vi "AVL Auto Time v0.1.vi"(9 "Time of Exit in":timestamp, 10 "Non-Auto Time in":dbl, 11 "State":T1) -> (2 "Time of Exit":timestamp, 3 "Non-Auto Time":dbl)   [LabVIEW 2021]
doc: "v0.1:\n- Added a state to reload values"
uses:
  Controls/AVL Auto Time.ctl
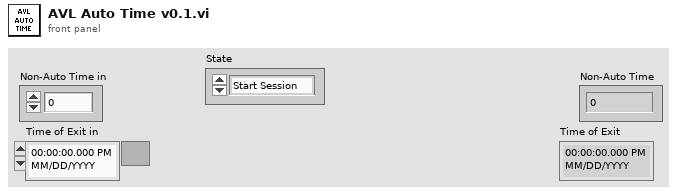
[diagram p1: front panel]
types:
  T1 = typedef "AVL Auto Time.ctl" = enum16{"Start Session", "Exited Auto", "Resumed Auto", "Read Time", "Reload Values"}
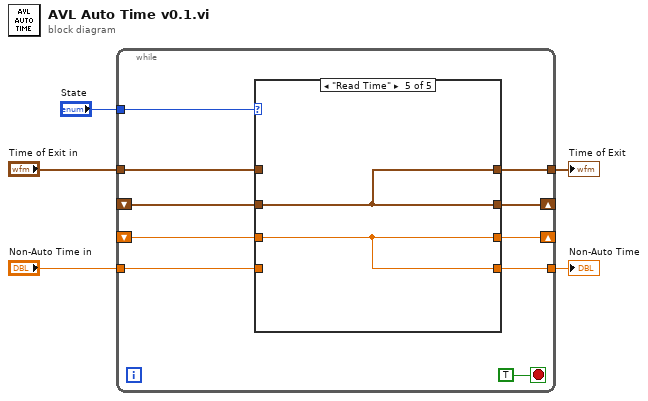
[diagram p0: block diagram]
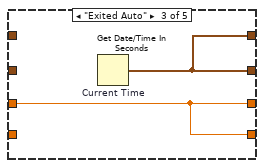
[diagram p4: hidden frame]
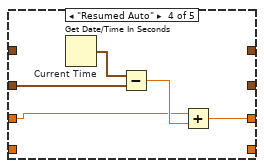
[diagram p5: hidden frame]
diagram:
  n1 = while {
    tunnel: "State" -> [w15]
    shift-right: [w14] -> _
    shift-left: _ -> [w13]
    shift-right: [w12] -> _
    shift-left: _ -> [w11]
    tunnel: [w10] -> w4
    tunnel: [w8] -> w3
    tunnel: "Time of Exit in" -> [w6]
    tunnel: "Non-Auto Time in" -> [w7]
    stop <- TRUE stop-if-true
    n2 = case shown="\"Read Time\"" w15 {
      tunnel: [_ w16 w18 _ w25] -> w14
      tunnel: w13 -> [_ _ _ w22 w25]
      tunnel: [_ w17 w19 w21 w26] -> w12
      tunnel: w11 -> [_ _ w19 w20 w26]
      tunnel: [_ _ w19 _ w26] -> w10
      tunnel: [_ _ w18 _ w25] -> w8
      tunnel: w7 -> [_ w17 _ _ _]
      tunnel: w6 -> [_ w16 _ _ _]
      frame "Start Session", Default {
      }
      frame "Reload Values" {
      }
      frame "Exited Auto" {
        n3 = Get Date/Time In Seconds "Current Time"() -> (seconds since 1Jan1904=w18:timestamp)
      }
      frame "Resumed Auto" {
        n4 = Get Date/Time In Seconds "Current Time"() -> (seconds since 1Jan1904=w24:timestamp)
        n5 = Subtract(x=w24, y=w22) -> (x-y=w23:dbl)
        n6 = Add(x=w20, y=w23) -> (x+y=w21:dbl)
      }
      frame "Read Time" {
      }
    }
  }
  "Non-Auto Time" <- w4
  "Time of Exit" <- w3
